vi "PXF4_get_current.vi"(8 "error in":errorcluster, 11 "Modbus Master in":refnum<class "Modbus Master.lvclass">) -> (0 "error out":errorcluster, 2 "A":dbl format="%.2f", 3 "Modbus Master out":refnum<class "Modbus Master.lvclass">)   [LabVIEW 2019]
uses:
  <vilib>/NI/Modbus Library/API/Master/Modbus Master.lvclass
panel:
  out "raw":u16
  out "register values":u16[](array[numeric])
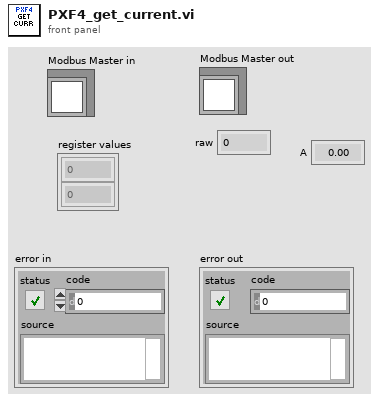
[diagram p1: front panel]
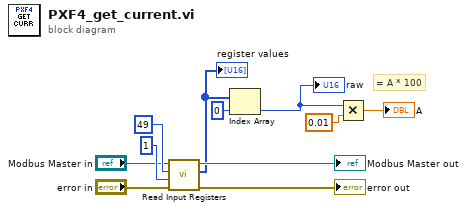
[diagram p0: block diagram]
diagram:
  # "= A * 100"
  n1 = call-dynamic "Read Input Registers.vi"("error in"="error in", "number of inputs"=u16 1, "starting address"=u16 49, "Modbus master in"="Modbus Master in") -> ("error out"=→"error out":errorcluster, "register values"=w8:u16[], "Modbus master out"=→"Modbus Master out":refnum<class "Modbus Master.lvclass">)  [unwired: 5 in]
  "register values" <- w8
  n2 = Index Array(array=w8, index=0) -> (element=w2:u16)
  "raw" <- w2
  n3 = Multiply(x=w2, y=0.01) -> (x*y=→"A":dbl)
